vi "RUN_VIS.vi"(5 "index":u8, 7 "arguments":string[](array[string]), 8 "dt":i32, 9 "Reinit":bool, 10 "bus_inputs":T1, 11 "bus_state":T2) -> (1 "Done":bool, 2 "bus_inputs out":T1, 3 "bus_state out":T2)   [LabVIEW 2013]
uses:
  structures/bus_state.ctl
  structures/bus_state_drivetrain.ctl
  structures/bus_state_collector.ctl
  collector/collector_shot_cal.ctl
  structures/bus_inputs.ctl
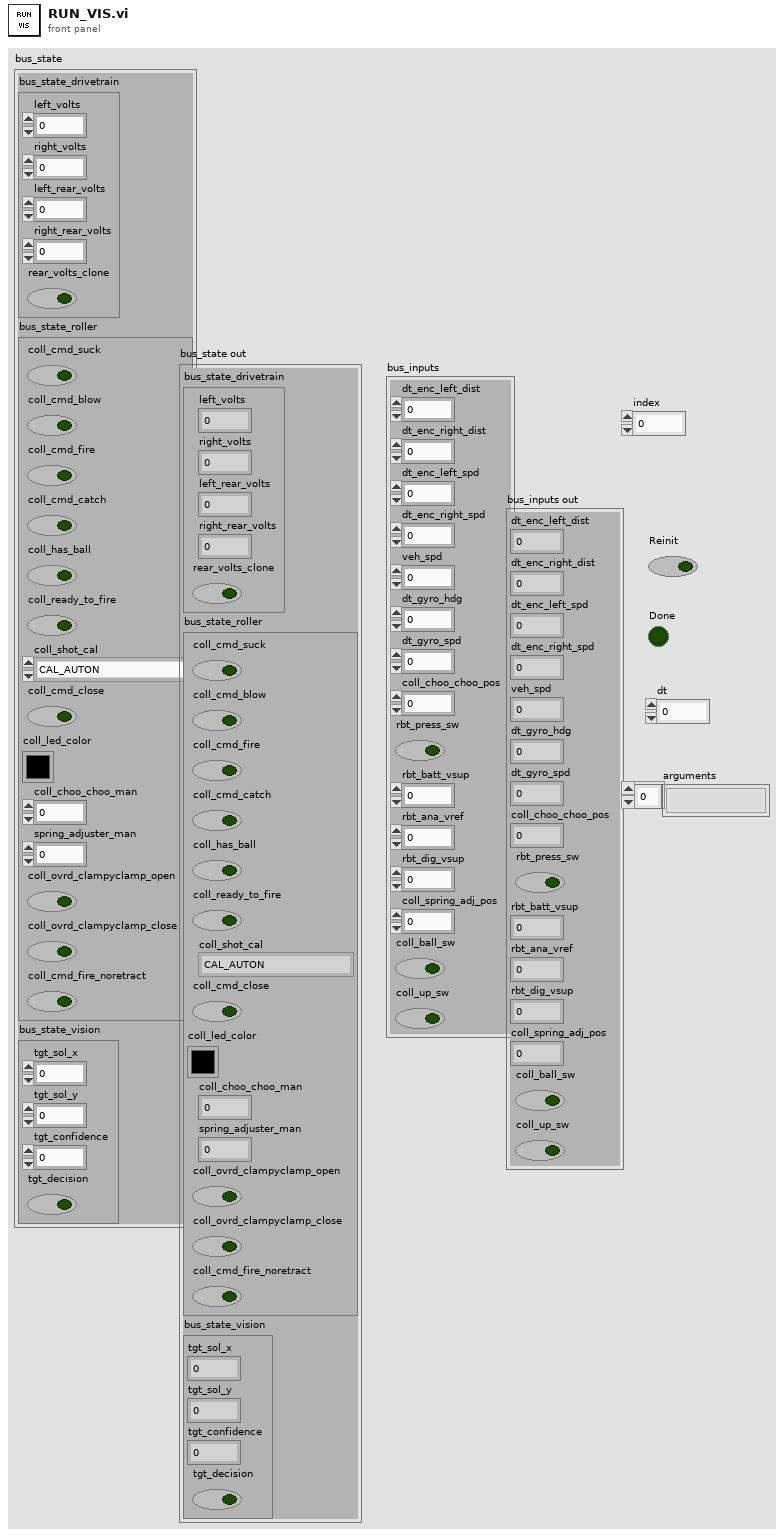
[diagram p1: front panel]
types:
  T1 = typedef "bus_inputs.ctl" = cluster{"dt_enc_left_dist":sgl, "dt_enc_right_dist":sgl, "dt_enc_left_spd":sgl, "dt_enc_right_spd":sgl, "veh_spd":sgl, "dt_gyro_hdg":sgl, "dt_gyro_spd":sgl, "coll_choo_choo_pos":sgl, "rbt_press_sw":bool, "rbt_batt_vsup":sgl, "rbt_ana_vref":dbl, "rbt_dig_vsup":dbl, "coll_spring_adj_pos":sgl, "coll_ball_sw":bool, "coll_up_sw":bool}
  T2 = typedef "bus_state.ctl" = cluster{"bus_state_drivetrain":T3, "bus_state_roller":T4, "bus_state_vision":cluster{"tgt_sol_x":dbl, "tgt_sol_y":dbl, "tgt_confidence":dbl, "tgt_decision":bool}}
  T3 = typedef "bus_state_drivetrain.ctl" = cluster{"left_volts":sgl, "right_volts":sgl, "left_rear_volts":sgl, "right_rear_volts":sgl, "rear_volts_clone":bool}
  T4 = typedef "bus_state_collector.ctl" = cluster{"coll_cmd_suck":bool, "coll_cmd_blow":bool, "coll_cmd_fire":bool, "coll_cmd_catch":bool, "coll_has_ball":bool, "coll_ready_to_fire":bool, "coll_shot_cal":T5, "coll_cmd_close":bool, "coll_led_color":u32, "coll_choo_choo_man":sgl, "spring_adjuster_man":sgl, "coll_ovrd_clampyclamp_open":bool, "coll_ovrd_clampyclamp_close":bool, "coll_cmd_fire_noretract":bool}
  T5 = typedef "collector_shot_cal.ctl" = enum16{"CAL_AUTON", "CAL_CLOSE", "CAL_MID", "CAL_FAR", "NOT_SAFE_TO_ACTUATE"}
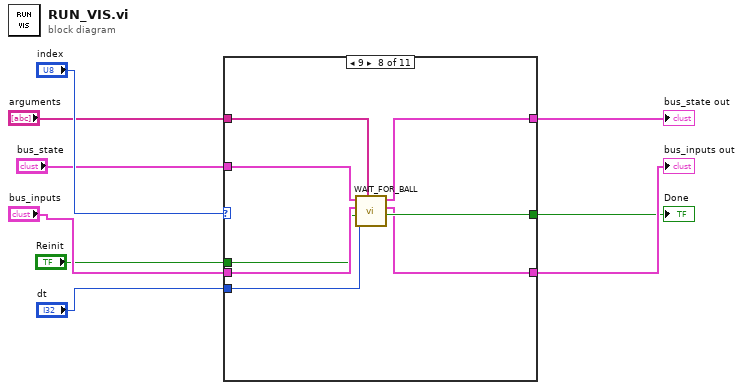
[diagram p0: block diagram]
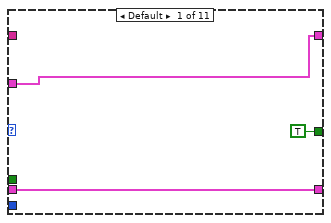
[diagram p2: hidden frame]
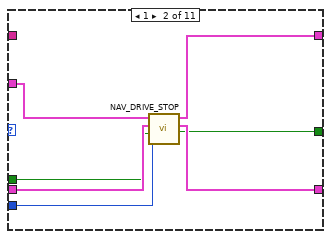
[diagram p3: hidden frame]
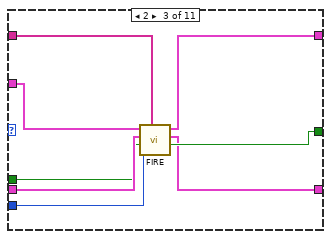
[diagram p4: hidden frame]
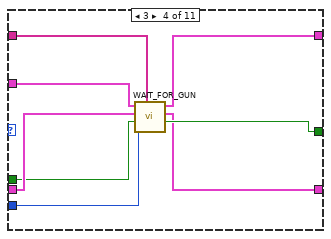
[diagram p5: hidden frame]
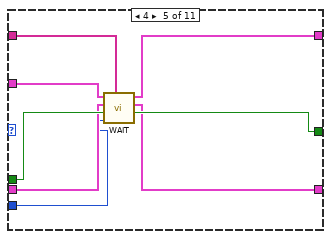
[diagram p6: hidden frame]
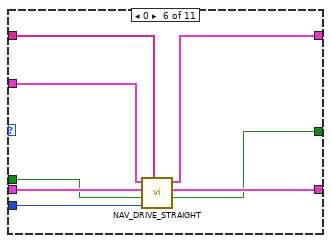
[diagram p7: hidden frame]
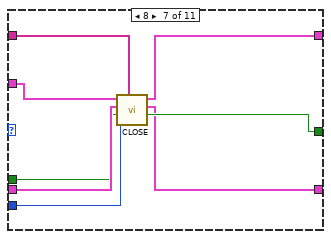
[diagram p8: hidden frame]
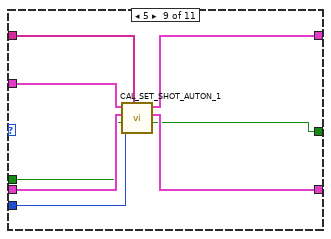
[diagram p9: hidden frame]
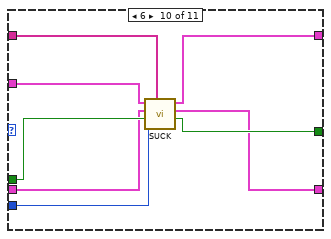
[diagram p10: hidden frame]
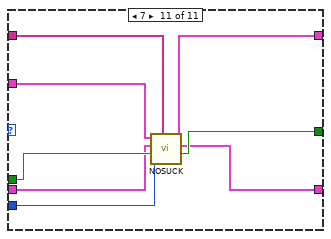
[diagram p11: hidden frame]
diagram:
  n1 = case shown="9" "index" {
    tunnel: "arguments" -> [_ _ w27 w34 w43 w51 w59 w66 w75 w83 w91]
    tunnel: "bus_state" -> [w12 w19 w26 w35 w42 w50 w58 w67 w74 w82 w90]
    tunnel: "bus_inputs" -> [w10 w15 w25 w33 w40 w49 w54 w62 w73 w80 w88]
    tunnel: "Reinit" -> [_ w13 w24 w32 w41 w48 w53 w61 w72 w81 w89]
    tunnel: "dt" -> [_ w14 w23 w31 w39 w47 w52 w60 w71 w79 w87]
    tunnel: [w12 w18 w22 w30 w38 w46 w57 w65 w70 w76 w85] -> w3
    tunnel: [w10 w17 w20 w28 w36 w45 w55 w63 w69 w77 w84] -> w2
    tunnel: [TRUE ("Done") w16 w21 w29 w37 w44 w56 w64 w68 w78 w86] -> w1
    frame Default {
    }
    frame 1 {
      n2 = call "NAV_DRIVE_STOP.vi"("dt"=w14, "Reinit"=w13, "bus_inputs"=w15, "bus_state"=w19) -> ("Done"=w16:bool, "bus_inputs out"=w17:T1, "bus_state out"=w18:T2)  [unwired: 5 in]
    }
    frame 2 {
      n3 = call "FIRE.vi"("arguments"=w27, "dt"=w23, "Reinit"=w24, "bus_inputs"=w25, "bus_state"=w26) -> ("Done"=w21:bool, "bus_inputs out"=w20:T1, "bus_state out"=w22:T2)  [unwired: 4 in]
    }
    frame 3 {
      n4 = call "WAIT_FOR_GUN.vi"("arguments"=w34, "dt"=w31, "Reinit"=w32, "bus_inputs"=w33, "bus_state"=w35) -> ("Done"=w29:bool, "bus_inputs out"=w28:T1, "bus_state out"=w30:T2)  [unwired: 4 in]
    }
    frame 4 {
      n5 = call "WAIT.vi"("arguments"=w43, "dt"=w39, "Reinit"=w41, "bus_inputs"=w40, "bus_state"=w42) -> ("Done"=w37:bool, "bus_inputs out"=w36:T1, "bus_state out"=w38:T2)  [unwired: 4 in]
    }
    frame 0 {
      n6 = call "NAV_DRIVE_STRAIGHT.vi"("arguments"=w51, "dt"=w47, "Reinit"=w48, "bus_inputs"=w49, "bus_state"=w50) -> ("Done"=w44:bool, "bus_inputs out"=w45:T1, "bus_state out"=w46:T2)  [unwired: 4 in]
    }
    frame 8 {
      n7 = call "CLOSE.vi"("arguments"=w59, "dt"=w52, "Reinit"=w53, "bus_inputs"=w54, "bus_state"=w58) -> ("Done"=w56:bool, "bus_inputs out"=w55:T1, "bus_state out"=w57:T2)  [unwired: 4 in]
    }
    frame 9 {
      n8 = call "WAIT_FOR_BALL.vi"("arguments"=w66, "dt"=w60, "Reinit"=w61, "bus_inputs"=w62, "bus_state"=w67) -> ("Done"=w64:bool, "bus_inputs out"=w63:T1, "bus_state out"=w65:T2)  [unwired: 4 in]
    }
    frame 5 {
      n9 = call "CAL_SET_SHOT_AUTON_1.vi"("arguments"=w75, "dt"=w71, "Reinit"=w72, "bus_inputs"=w73, "bus_state"=w74) -> ("Done"=w68:bool, "bus_inputs out"=w69:T1, "bus_state out"=w70:T2)  [unwired: 4 in]
    }
    frame 6 {
      n10 = call "SUCK.vi"("arguments"=w83, "dt"=w79, "Reinit"=w81, "bus_inputs"=w80, "bus_state"=w82) -> ("Done"=w78:bool, "bus_inputs out"=w77:T1, "bus_state out"=w76:T2)  [unwired: 4 in]
    }
    frame 7 {
      n11 = call "NOSUCK.vi"("arguments"=w91, "dt"=w87, "Reinit"=w89, "bus_inputs"=w88, "bus_state"=w90) -> ("Done"=w86:bool, "bus_inputs out"=w84:T1, "bus_state out"=w85:T2)  [unwired: 4 in]
    }
  }
  "bus_state out" <- w3
  "bus_inputs out" <- w2
  "Done" <- w1
